vi "Get Default Actor Class Path.vi"(8 "error in (no error)":errorcluster, 11 "Actor Store":refnum<class "Actor Store.lvclass">) -> (0 "error out":errorcluster, 1 "Actor Label":string, 2 "Path String":path, 3 "Actor Store":refnum<class "Actor Store.lvclass">)   [LabVIEW 2020, in "Add Actor.lvlib"]
uses:
  Add Actor.lvlib
  Classes/Actor Store/Actor Store.lvclass
  <vilib>/Utility/LVLibp/NI_PackedLibraryUtility.lvlib
  MessageMakerProvider/AFPP Shared/AFPP Shared.lvlib
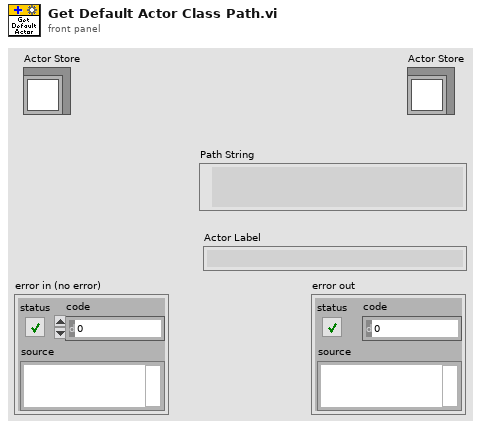
[diagram p1: front panel]
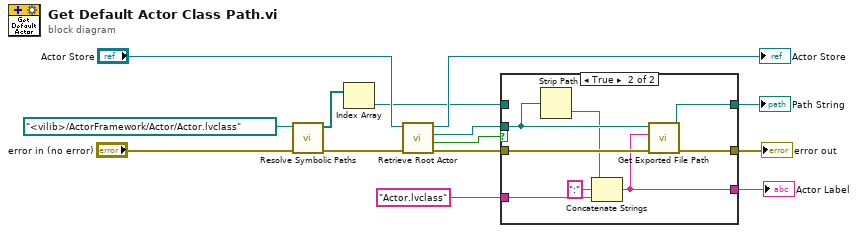
[diagram p0: block diagram]
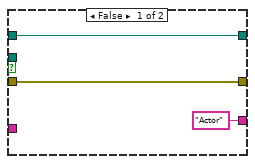
[diagram p2: hidden frame]
diagram:
  n1 = call "Resolve Symbolic Paths.vi"("error in (no error)"="error in (no error)", "Path"=path "<vilib>/ActorFramework/Actor/Actor.lvclass") -> ("error out"=w4:errorcluster, "Resolved Paths"=w2:path[])  [unwired: 8 in]
  n2 = Index Array(array=w2) -> (element=w1:path)  [unwired: 1 in]
  n3 = call-dynamic "Retrieve Root Actor.vi"("error in (no error)"=w4, "Actor Store in"="Actor Store") -> ("error out"=w13:errorcluster, "valid?"=w12:bool, "Root Actor"=w14:path, "Actor Store out"=→"Actor Store":refnum<class "Actor Store.lvclass">)  [unwired: 6 in]
  n4 = case shown="True" w12 {
    tunnel: w13 -> [w17 w25]
    tunnel: [w17 w23] -> w9
    tunnel: w1 -> [w16 _]
    tunnel: [w16 w24] -> w11
    tunnel: w14 -> [_ w21]
    tunnel: "Actor.lvclass" ("qualified name") -> [_ w22]
    tunnel: ["Actor" w18] -> w8
    frame False {
    }
    frame True {
      n5 = Strip Path(path=w21) -> (name=w20:string)  [unwired: 1 out]
      n6 = Concatenate Strings(w20, ":" ("string"), w22) -> (w18:string)
      n7 = call <vilib>:"Get Exported File Path.vi"("error in (no error)"=w25, "qualified name"=w18, "packed library path"=w21) -> ("error out"=w23:errorcluster, "path"=w24:path)  [unwired: 7 in]
    }
  }
  "error out" <- w9
  "Path String" <- w11
  "Actor Label" <- w8
